vi "十六进制字符串至普通字符串转换(个人编写).vi"(1 "十六进制字符串":string) -> (0 "普通字符串":string)   [LabVIEW 2012]
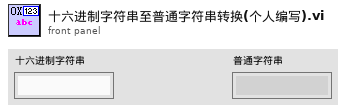
[diagram p1: front panel]
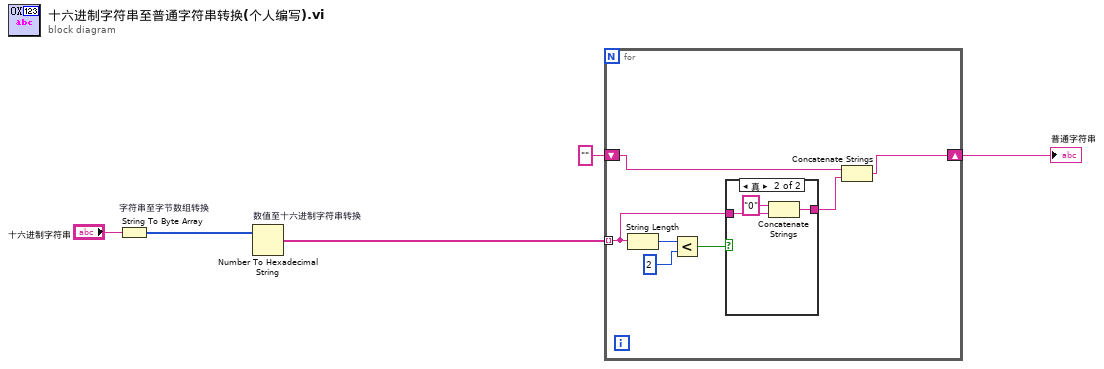
[diagram p0: block diagram]
diagram:
  n1 = String To Byte Array "字符串至字节数组转换"(string="十六进制字符串") -> (unsigned byte array=w5:u8[])
  n2 = Number To Hexadecimal String "数值至十六进制字符串转换"(2:w5) -> (0:w3:string[])  [unwired: 1 in]
  n3 = for {
    tunnel: w3 -> [w7] mode=indexing
    shift-right: [w11] -> w1
    shift-left: "" -> [w12]
    n4 = String Length(string=w7) -> (length=w10:i32)
    n5 = Less?(x=w10, y=2) -> (x < y?=w8:bool)
    n6 = case shown="真" w8 {
      tunnel: w7 -> [w13 w16]
      tunnel: [w13 w14] -> w6
      frame False {
      }
      frame True {
        n7 = Concatenate Strings("0" ("字符串"), w16) -> (w14:string)
      }
    }
    n8 = Concatenate Strings(w12, w6) -> (w11:string)
  }
  "普通字符串" <- w1
